vi "Constructor.vi"(8 "error in (no error)":errorcluster) -> (0 "error out":errorcluster, 3 "_IconEditorInterface out":refnum<class "_IconEditorInterface.lvclass">)   [LabVIEW 2021, in "_IconEditorInterface.lvlib" / "_IconEditorInterface.lvclass"]
uses:
  _IconEditorInterface.lvclass
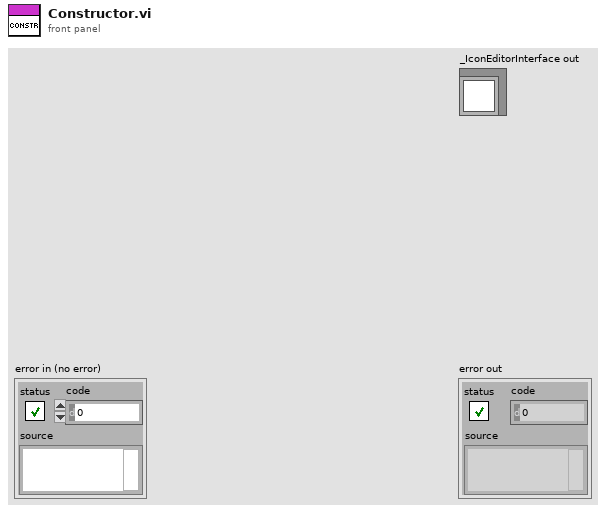
[diagram p1: front panel]
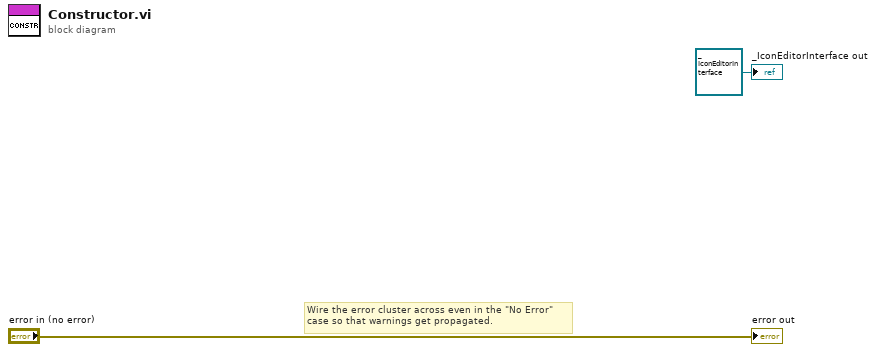
[diagram p0: block diagram]
diagram:
  # "Wire the error cluster across even in the \"No Error\"\ncase so that warnings get propagated."
  "error out" <- "error in (no error)"
  "_IconEditorInterface out" <- refnum<class "_IconEditorInterface.lvclass"> refnum ("_IconEditorInterface out")
